vi "Update Core.vi"(8 "error in (no error)":errorcluster, 11 "Level Controller in":refnum<class "Level Controller.lvclass">) -> (0 "error out":errorcluster, 3 "Level Controller out":refnum<class "Level Controller.lvclass">)   [LabVIEW 2025, in "Level Controller.lvlib" / "Level Controller.lvclass"]
doc: "Child classes should NOT override this VI. This VI is defined by the Timed Loop Actor parent class. In this level controller, the update behavior is to check the variable that the level controller monitors and execute a change of state depending upon whether or not the variable is above or below the deadband range."
uses:
  Level Controller.lvclass
  Level Controller.lvclass/Level Controller.ctl
  Value Position.ctl
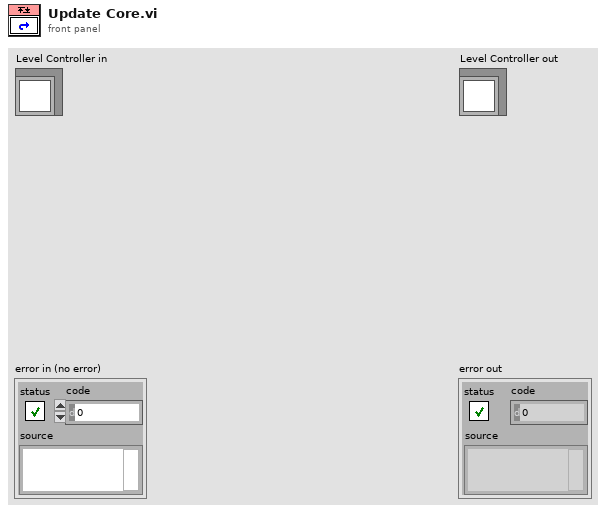
[diagram p1: front panel]
types:
  T1 = typedef "Level Controller.lvlib/Level Controller.lvclass/Value Position.ctl" = enum16{"Never Assigned", "Above Level", "Below Level"}
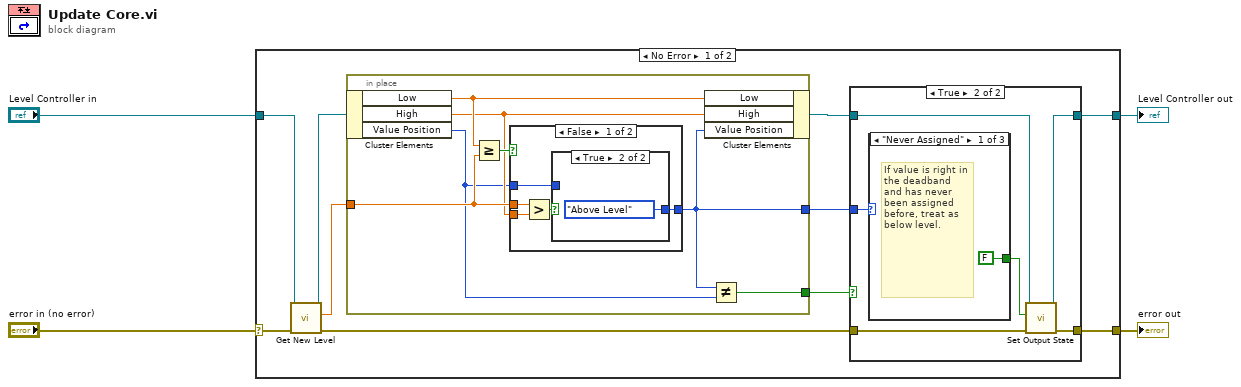
[diagram p0: block diagram]
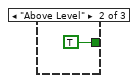
[diagram p3: hidden frame]
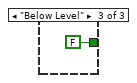
[diagram p4: hidden frame]
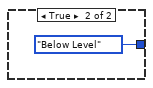
[diagram p6: hidden frame]
diagram:
  n1 = case shown="No Error" "error in (no error)" {
    selector: "error in (no error)" -> [w14 w42]
    tunnel: [w13 w42] -> w3
    tunnel: [w8 w41] -> w2
    tunnel: "Level Controller in" -> [w10 w41]
    frame No Error {
      n2 = call-dynamic "Get New Level.vi"("error in (no error)"=w14, "Level Controller in"=w10) -> ("error out"=w12:errorcluster, "Level"=w11:dbl, "Level Controller out"=w5:refnum<class "Level Controller.lvclass">)  [unwired: 7 in]
      n3 = in-place {
        in-place-border: w11 -> [w30]
        in-place-border: [w32] -> w7
        in-place-border: [w27] -> w6
        n4 = in-place-cluster #1(w5) -> ("Low"=w31:dbl, "High"=w28:dbl, "Value Position"=w26:T1)
        n5 = Greater Or Equal?(x=w31, y=w30) -> (x >= y?=w29:bool)
        n6 = case shown="False" w29 {
          tunnel: w30 -> [w37 _]
          tunnel: [w35 Value_Position."Below Level" ("Value Position")] -> w27
          tunnel: w28 -> [w36 _]
          tunnel: w26 -> [w33 _]
          frame False {
            n7 = Greater?(x=w37, y=w36) -> (0:w34:bool)
            n8 = case shown="True" w34 {
              tunnel: [w38 Value_Position."Above Level" ("Value Position")] -> w35
              tunnel: w33 -> [w38 _]
              frame False {
              }
              frame True {
              }
            }
          }
          frame True {
          }
        }
        n9 = in-place-cluster #1("Low"=w31, "High"=w28, "Value Position"=w27) -> (w9:refnum<class "Level Controller.lvclass">)
        n10 = Not Equal?(x=w27, y=w26) -> (x != y?=w32:bool)
      }
      n11 = case shown="True" w7 {
        tunnel: [w15 w22] -> w13
        tunnel: w12 -> [w15 w21]
        tunnel: w9 -> [w16 w20]
        tunnel: [w16 w19] -> w8
        tunnel: w6 -> [_ w18]
        frame False {
        }
        frame True {
          n12 = case shown="\"Never Assigned\"" w18 {
            tunnel: [FALSE TRUE FALSE] -> w17
            frame "Never Assigned" {
              # "If value is right in the deadband and has never been assigned before, treat as below level."
            }
            frame "Above Level" {
            }
            frame "Below Level" {
            }
          }
          n13 = call-dynamic "Set Output State.vi"("error in (no error)"=w21, "Output State"=w17, "Level Controller in"=w20) -> ("error out"=w22:errorcluster, "Level Controller out"=w19:refnum<class "Level Controller.lvclass">)  [unwired: 7 in]
        }
      }
    }
    frame Error {
    }
  }
  "error out" <- w3
  "Level Controller out" <- w2
